vi "InstrParam.vi"(4 "queue out":refnum<queue>, 6 "user event out":refnum<user-event>, 8 "error in (no error)":errorcluster caption="entrée d'erreur (pas d'erreur)", 10 "InstrParam":string, 11 "BaseDevice en entrée":refnum<class "BaseDevice.lvclass"> caption="DNL_LabVIEW Object in") -> (0 "error out":errorcluster caption="sortie d'erreur", 3 "BaseDevice en sortie":refnum<class "BaseDevice.lvclass"> caption="DNL_LabVIEW Object out")   [LabVIEW 2019, in "BaseDevice.lvclass"]
uses:
  BaseDevice.lvclass
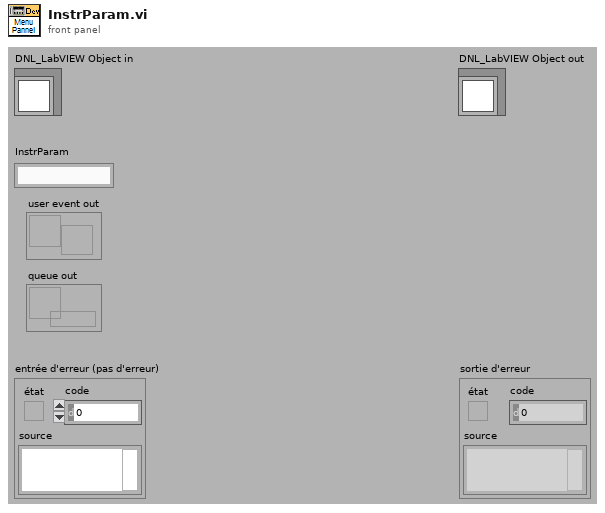
[diagram p1: front panel]
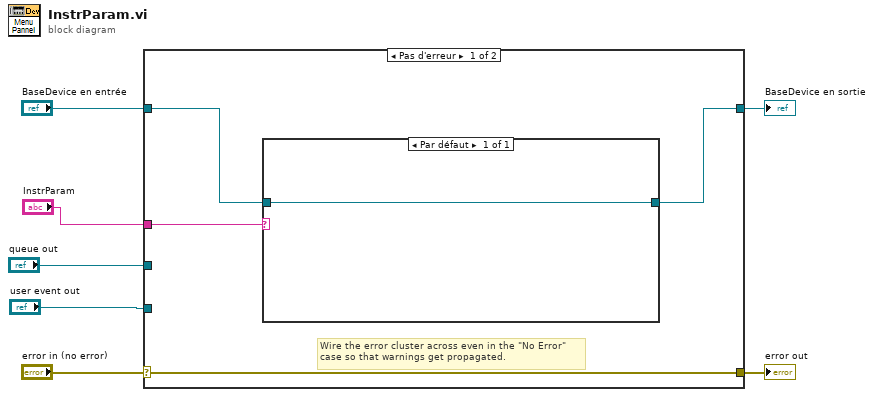
[diagram p0: block diagram]
diagram:
  n1 = case shown="Pas d'erreur" "error in (no error)" {
    selector: "error in (no error)" -> [w11 w14]
    tunnel: [w11 w14] -> w6
    tunnel: [w8 w13] -> w4
    tunnel: "BaseDevice en entrée" -> [w9 w13]
    tunnel: "InstrParam" -> [w10 _]
    tunnel: "queue out" -> [_ _]
    tunnel: "user event out" -> [_ _]
    frame No Error {
      # "Wire the error cluster across even in the \"No Error\"\ncase so that warnings get propagated."
      n2 = case shown="Par défaut" w10 {
        tunnel: [w12] -> w8
        tunnel: w9 -> [w12]
        frame Par défaut {
        }
      }
    }
    frame Error {
    }
  }
  "error out" <- w6
  "BaseDevice en sortie" <- w4
